vi "MorphologyCore.vi"(5 "MorphologyType":T1, 6 "Iterations":u16, 7 "Anchor Point":T2={"x"=-1, "y"=-1}, 8 "error in (no error)":errorcluster, 9 "Structuring Element":bool[][](array[boolean]), 11 "Greyscale Image-Source in":T3) -> (0 "error out":errorcluster)   [LabVIEW 2020, in "image.lvlib"]
uses:
  image.lvlib
  Greyscale Image.ctl
  common/Image Point (Integer).ctl
  MorphologyTypes.ctl
  common/common.lvlib
  common/bin/gartoolkit_32-1.dll
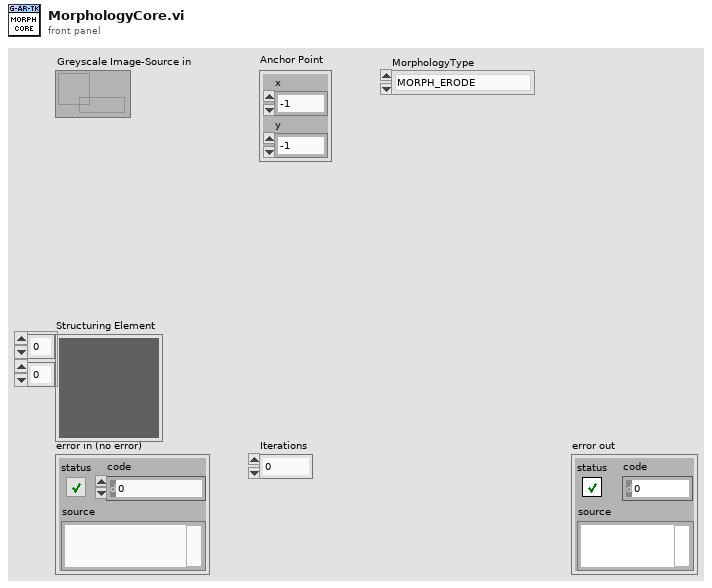
[diagram p1: front panel]
types:
  T1 = typedef "image.lvlib/MorphologyTypes.ctl" = enum16{"MORPH_ERODE", "MORPH_DILATE", "MORPH_OPEN", "MORPH_CLOSE", "MORPH_GRADIENT", "MORPH_TOPHAT", "MORPH_BLACKHAT", "MORPH_HITMISS"}
  T2 = typedef "common.lvlib/Image Point (Integer).ctl" = cluster{"x":i32, "y":i32}
  T3 = typedef "image.lvlib/Greyscale Image.ctl" = refnum<data-value>
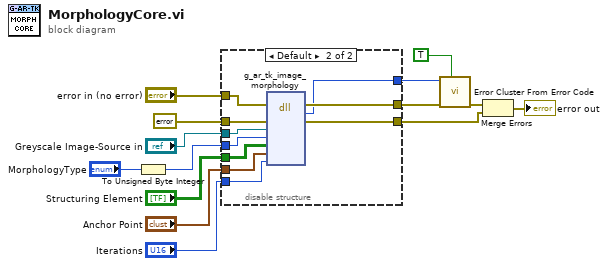
[diagram p0: block diagram]
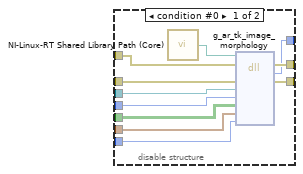
[diagram p2: hidden frame]
diagram:
  n1 = To Unsigned Byte Integer(number="MorphologyType") -> (unsigned 8bit integer=w8:u8)
  n2 = disable-structure shown="Default" {
    disable-tunnel: "error in (no error)" -> [w25 w35]
    disable-tunnel: errorcluster {"status"=FALSE, "code"=0, "source"=""} ("error constant") -> [w24 w34]
    disable-tunnel: "Greyscale Image-Source in" -> [w23 w33]
    disable-tunnel: w8 -> [w22 w32]
    disable-tunnel: "Structuring Element" -> [w21 w31]
    disable-tunnel: "Anchor Point" -> [w20 w30]
    disable-tunnel: "Iterations" -> [w19 w29]
    disable-tunnel: [w18 w28] -> w4
    disable-tunnel: [w17 w27] -> w3
    disable-tunnel: [w16 w26] -> w2
    frame condition #0 {
      n3 = call "NI-Linux-RT Shared Library Path (Core).vi"() -> ("Path"=w15:path)
      n4 = dll-call lib="?" fn="g_ar_tk_image_morphology" ("g_ar_toolkit.*.*:g_ar_tk_image_in_range")(path in=w15, error in=w25, "error_cluster"=w24, "EDVR src"=w23, "operation"=w22, "kernel"=w21, "anchor_point"=w20, "iterations"=w19) -> (error out=w18:errorcluster, w17:i32, "error_cluster"=w16:errorcluster)  [unwired: 6 in, 1 out]
    }
    frame condition #1 (active) {
      n5 = dll-call lib="C:/serenial/lib/g-augmented-reality-toolkit/LabVIEW/common/bin/gartoolkit_*-1.*" fn="g_ar_tk_image_morphology" ("g_ar_toolkit.*.*:g_ar_tk_image_in_range")(error in=w35, "error_cluster"=w34, "EDVR src"=w33, "operation"=w32, "kernel"=w31, "anchor_point"=w30, "iterations"=w29) -> (error out=w28:errorcluster, w27:i32, "error_cluster"=w26:errorcluster)  [unwired: 7 in, 1 out]
    }
  }
  n6 = call <vilib>:"Error Cluster From Error Code.vi"("show call chain? (False)"=TRUE, "error in (no error)"=w4, "error code (0)"=w3) -> ("error out"=w13:errorcluster)  [unwired: 6 in]
  n7 = Merge Errors(w13, w2) -> (→"error out":errorcluster)
